vi "PKG_IMC_InitCfg.vi"(11 "handle":u32) -> (2 "function return":i32, 3 "handle out":u32)   [LabVIEW 2011, in "IMC_Pkg4xxx.lvlib"]
doc: "IMC_PKG_API int WINAPI PKG_IMC_InitCfg(IMC_HANDLE handle);"
uses:
  IMC_Pkg4xxx.lvlib
  IMC_Pkg4xxx.dll
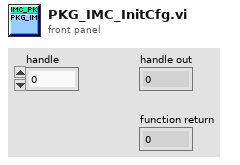
[diagram p1: front panel]
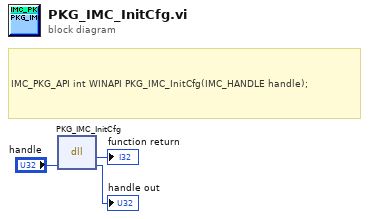
[diagram p0: block diagram]
diagram:
  # "IMC_PKG_API int WINAPI PKG_IMC_InitCfg(IMC_HANDLE handle);"
  n1 = dll-call lib="PTH1mabs F光盘刻录\niMC MotionIMCNet_V4.0IMCAppincLabviewIMC_PKG4xxxIMC_PKG4xxx\nIMC_Pkg4xxx.*" fn="PKG_IMC_InitCfg"("handle"="handle") -> (→"function return":i32, "handle"=→"handle out":u32)  [unwired: 3 in, 2 out]
